vi "纳清pH_所有参数读取.vi"(8 "error in (no error)":errorcluster caption="错误输入（无错误）", 11 "MB session in":refnum<class "MB_Master.lvclass">) -> (0 "error out":errorcluster caption="错误输出", 2 "输出值":T1 {"波特率" items=["4800", "9600", "19200", "38400", "57600", "115200"]}, 3 "MB session out":refnum<class "MB_Master.lvclass">)   [LabVIEW 2016, in "斯坦道多参数.lvlib"]
uses:
  <vilib>/Plasmionique/MB Master/MB_Master/MB_Master.lvclass
  <vilib>/Plasmionique/MB Master/MB Master.lvlib
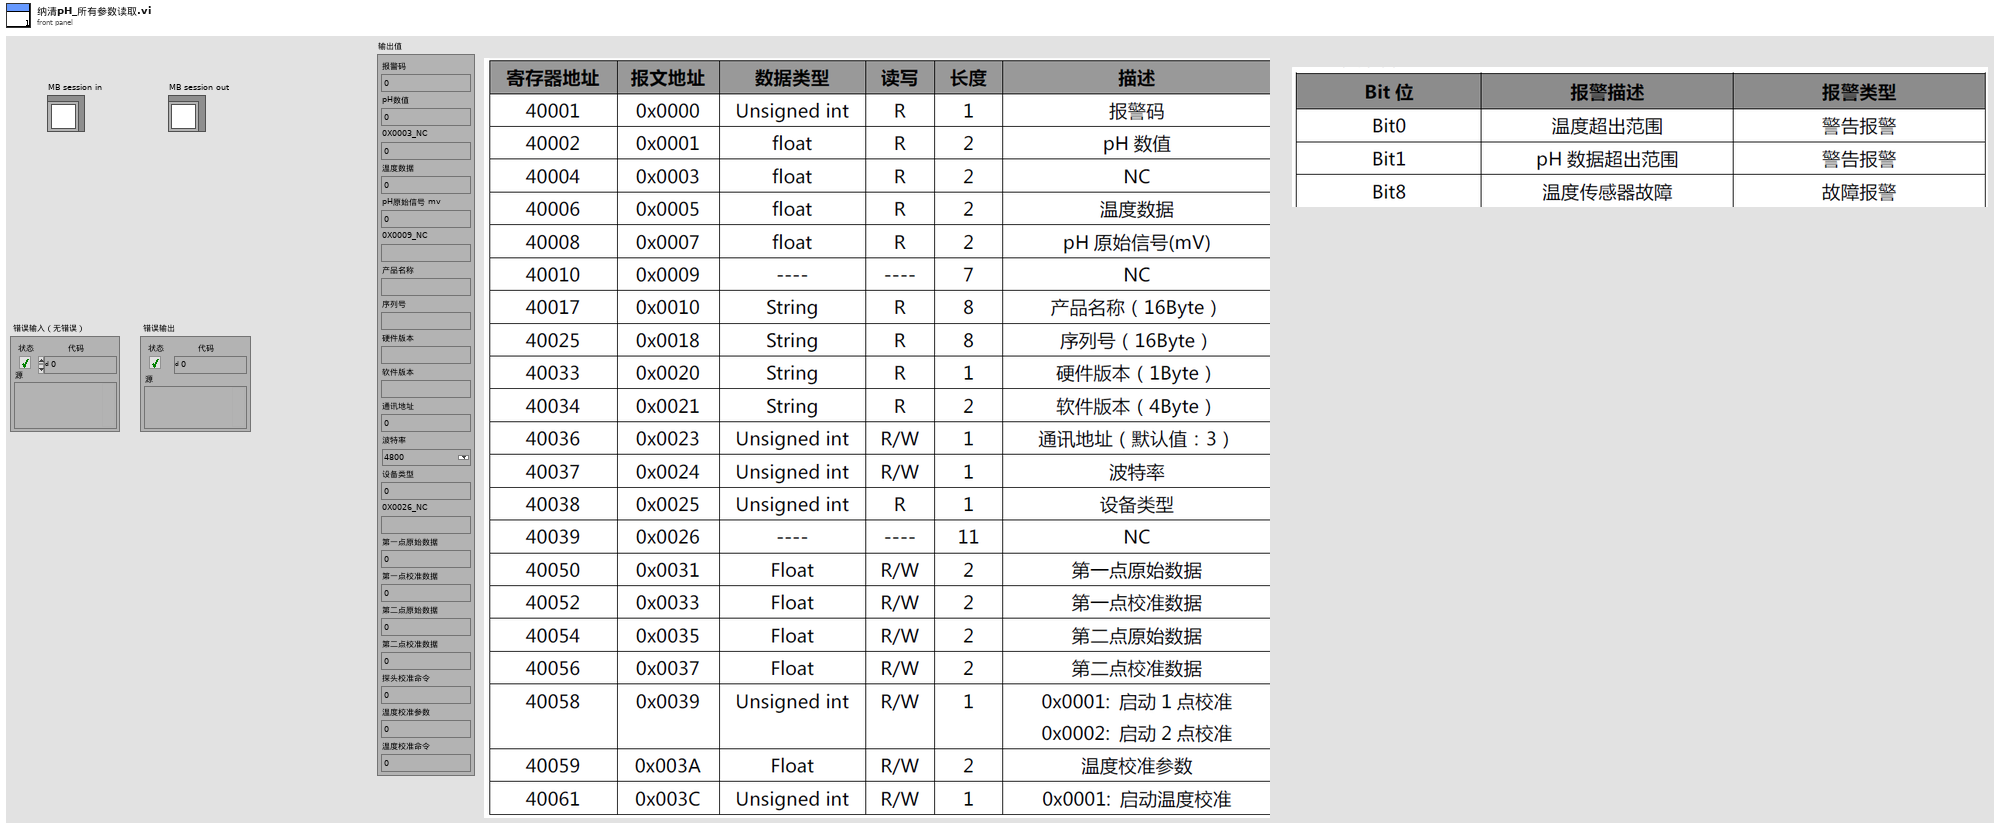
[diagram p1: front panel]
types:
  T1 = cluster{"报警码":u16, "pH数值":sgl, "0X0003_NC":sgl, "温度数据":sgl, "pH原始信号 mv":sgl, "0X0009_NC":string, "产品名称":string, "序列号":string, "硬件版本":string, "软件版本":string, "通讯地址":u16, "波特率":u16, "设备类型":u16, "0X0026_NC":string, "第一点原始数据":sgl, "第一点校准数据":sgl, "第二点原始数据":sgl, "第二点校准数据":sgl, "探头校准命令":u16, "温度校准参数":sgl, "温度校准命令":u16}
  T2 = cluster{u16, "mode":dbl, "数值":sgl, "数值":sgl, "数值":sgl, "类型":string, "类型":string, "类型":string, "类型":string, "类型":string, u16, u16, u16, "类型":string, "数值":sgl, "数值":sgl, "数值":sgl, "数值":sgl, u16, "数值":sgl, u16}
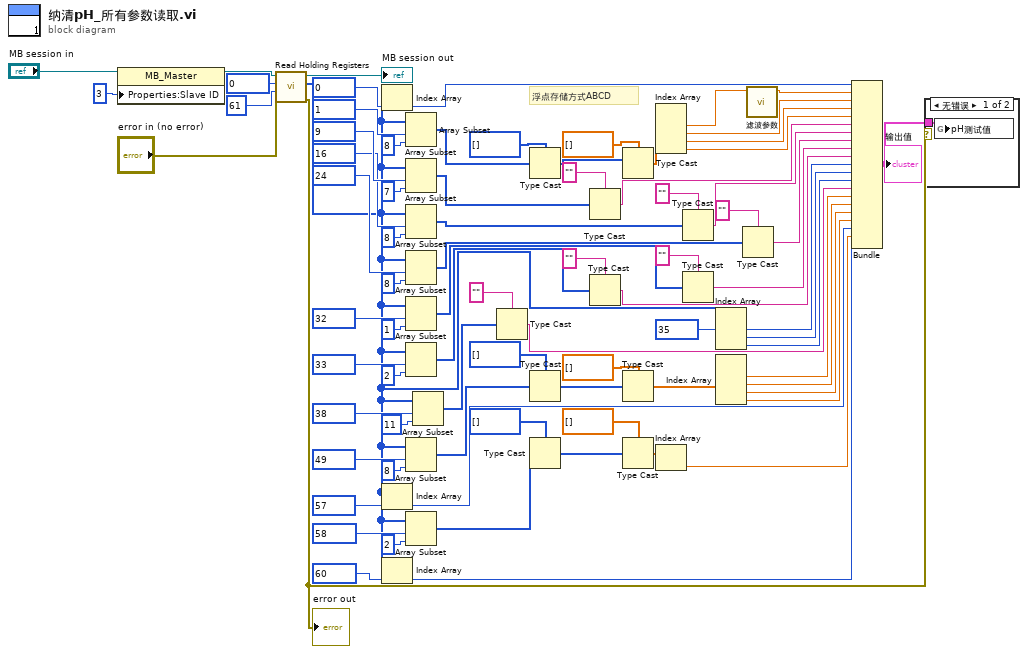
[diagram p0: block diagram]
diagram:
  # "浮点存储方式ABCD"
  n1 = property class="MB_Master"(reference="MB session in", "Properties:Slave ID"=u8 3 ("Slave ID")) -> (reference out=w71:refnum<class "MB_Master.lvclass">)  [unwired: 1 in, 1 out]
  n2 = call <vilib>:"Read Holding Registers.vi"("error in (no error)"="error in (no error)", "quantity"=u16 61, "starting address"=u16 0, "MB session in"=w71) -> ("error out"=w12:errorcluster, "Registers"=w14:u16[], "MB session out"=→"MB session out":refnum<class "MB_Master.lvclass">)  [unwired: 5 in]
  "error out" <- w12
  n3 = Index Array(array=w14, index=u16 0 ("starting address")) -> (element=w79:u16)
  n4 = Index Array(array=w14, index=u16 57 ("starting address")) -> (element=w17:u16)
  n5 = Index Array(array=w14, index=u16 60 ("starting address")) -> (element=w13:u16)
  n6 = Array Subset(array=w14, index=u16 1 ("starting address"), length=8 ("长度")) -> (w75:u16[])
  n7 = Array Subset(array=w14, index=u16 9 ("starting address"), length=7 ("长度")) -> (w65:u16[])
  n8 = Array Subset(array=w14, index=u16 16 ("starting address"), length=8 ("长度")) -> (w61:u16[])
  n9 = Array Subset(array=w14, index=u16 24 ("starting address"), length=8 ("长度")) -> (w55:u16[])
  n10 = Array Subset(array=w14, index=u16 32 ("starting address"), length=1 ("长度")) -> (w51:u16[])
  n11 = Array Subset(array=w14, index=u16 33 ("starting address"), length=2 ("长度")) -> (w45:u16[])
  n12 = Array Subset(array=w14, index=u16 49 ("starting address"), length=8 ("长度")) -> (w32:u16[])
  n13 = Array Subset(array=w14, index=u16 58 ("starting address"), length=2 ("长度")) -> (w20:u16[])
  n14 = Array Subset(array=w14, index=u16 38 ("starting address"), length=11 ("长度")) -> (w35:u16[])
  n15 = Type Cast(type="" ("类型"), x=w35) -> (*(type *) &x=w34:string)
  n16 = Type Cast(type=u32[] [] ("数组 2"), x=w75) -> (*(type *) &x=w11:u32[])
  n17 = Type Cast(type=u32[] [] ("数组 2"), x=w32) -> (*(type *) &x=w30:u32[])
  n18 = Type Cast(type=u32[] [] ("数组 2"), x=w20) -> (*(type *) &x=w22:u32[])
  n19 = Type Cast(type="" ("类型"), x=w65) -> (*(type *) &x=w63:string)
  n20 = Type Cast(type="" ("类型"), x=w45) -> (*(type *) &x=w43:string)
  n21 = Type Cast(type=sgl[] [] ("数组 2"), x=w11) -> (*(type *) &x=w74:sgl[])
  n22 = Type Cast(type=sgl[] [] ("数组 2"), x=w30) -> (*(type *) &x=w27:sgl[])
  n23 = Type Cast(type=sgl[] [] ("数组 2"), x=w22) -> (*(type *) &x=w25:sgl[])
  n24 = Index Array(array=w74) -> (element #1=w2:sgl, element #2=w69:sgl, element #3=w8:sgl, element #4=w7:sgl)  [unwired: 4 in]
  n25 = Index Array(array=w25) -> (element=w16:sgl)  [unwired: 1 in]
  n26 = Type Cast(type="" ("类型"), x=w61) -> (*(type *) &x=w58:string)
  n27 = Type Cast(type="" ("类型"), x=w51) -> (*(type *) &x=w48:string)
  n28 = Index Array(array=w14, index #1=u16 35 ("starting address")) -> (element #1=w41:u16, element #2=w40:u16, element #3=w39:u16)  [unwired: 2 in]
  n29 = Index Array(array=w27) -> (element #1=w26:sgl, element #2=w6:sgl, element #3=w5:sgl, element #4=w4:sgl)  [unwired: 4 in]
  n30 = Type Cast(type="" ("类型"), x=w55) -> (*(type *) &x=w53:string)
  n31 = call "滤波参数.vi"("x"=w2) -> ("mode"=w1:dbl)  [unwired: 10 in]
  n32 = Bundle(w79, "mode"=w1, "数值"=w69, "数值"=w8, "数值"=w7, "类型"=w63, "类型"=w58, "类型"=w53, "类型"=w48, "类型"=w43, w41, w40, w39, "类型"=w34, "数值"=w26, "数值"=w6, "数值"=w5, "数值"=w4, w17, "数值"=w16, w13) -> (w3:T2)  [unwired: 1 in]
  "输出值" <- w3
  n33 = case shown="无错误" w12 {
    tunnel: w3 -> [w82 _]
    frame No Error {
      n34 = global write "纳清过程全局变量.vi" "pH测试值"(w82) -> ()
    }
    frame Error {
    }
  }
